vi "Get Position Data.vi"(8 "error in (no error)":errorcluster, 10 "Complete NMEA Sentences":string[](array[string]), 11 "VISA resource name":refnum<visa-resource-name>) -> (0 "error out":errorcluster, 1 "Position Data":T1(array[cluster]), 2 "Complete NMEA Sentences (Copy)":string[](array[string]), 3 "VISA resource name out":refnum<visa-resource-name>)   [LabVIEW 2011, in "u-blox 5 Series.lvlib"]
doc: "Parses out the position data from all of the sentences that Read Raw.vi outputs, and passes through a complete copy of those sentences. Can be used in conjunction with other advanced \"Get\" VIs. See u-blox 5 Series Acquire and Chart GPS Advanced.vi for an example of how to use this VI.\n\nNote that the VISA Resource is not required, since this VI is a helper that does not actually interact with the device. The VISA Resource can be used, however, to clarify programming and maintain uniformity."
uses:
  u-blox 5 Series.lvlib
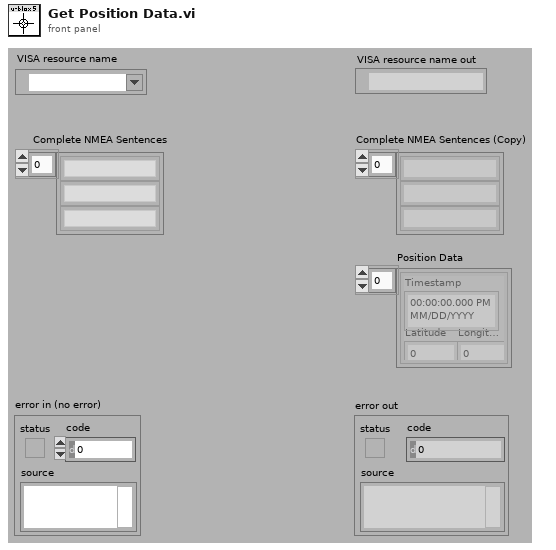
[diagram p1: front panel]
types:
  T1 = cluster{"Timestamp":timestamp, "Latitude":dbl, "Longitude":dbl}[]
  T2 = cluster{"Timestamp":timestamp, "Latitude":dbl, "Longitude":dbl}
  T3 = typedef "u-blox 5 Series.lvlib/GGA Data.ctl" = cluster{"time of fix":cluster{"included?":bool, "time":timestamp}, "latitude":cluster{"included?":bool, "latitude (deg)":dbl}, "longitude":cluster{"included?":bool, "longitude (deg)":dbl}, "fix quality":cluster{"included?":bool, "quality":u16}, "number of satellites in view":cluster{"included?":bool, "number of satellites":i8}, "horizontal dilution of precision":cluster{"included?":bool, "horizontal DOP":dbl}, "altitude above mean sea level":cluster{"included?":bool, "altitude (m)":dbl}, "height of geoid above WGS84":cluster{"included?":bool, "height of geoid (m)":dbl}, "time since last DGPS update":cluster{"included?":bool, "time (s)":dbl}, "DGPS station ID number":cluster{"included?":bool, "station ID number":dbl}}
  T4 = typedef "u-blox 5 Series.lvlib/RMC Data.ctl" = cluster{"time of fix":cluster{"included?":bool, "time":timestamp}, "status":cluster{"included?":bool, "value":u16}, "latitude":cluster{"included?":bool, "latitude (deg)":dbl}, "longitude":cluster{"included?":bool, "longitude (deg)":dbl}, "ground speed":cluster{"included?":bool, "speed (knots)":dbl}, "true track angle":cluster{"included?":bool, "angle (deg)":dbl}, "magnetic variation":cluster{"included?":bool, "variation (deg)":dbl}, "type of fix":cluster{"included?":bool, "mode":u16}}
  T5 = typedef "u-blox 5 Series.lvlib/GLL Data.ctl" = cluster{"latitude":cluster{"included?":bool, "latitude (deg)":dbl}, "longitude":cluster{"included?":bool, "longitude (deg)":dbl}, "time of fix":cluster{"included?":bool, "time":timestamp}, "status":cluster{"included?":bool, "value":u16}, "type of fix":cluster{"included?":bool, "mode":u16}}
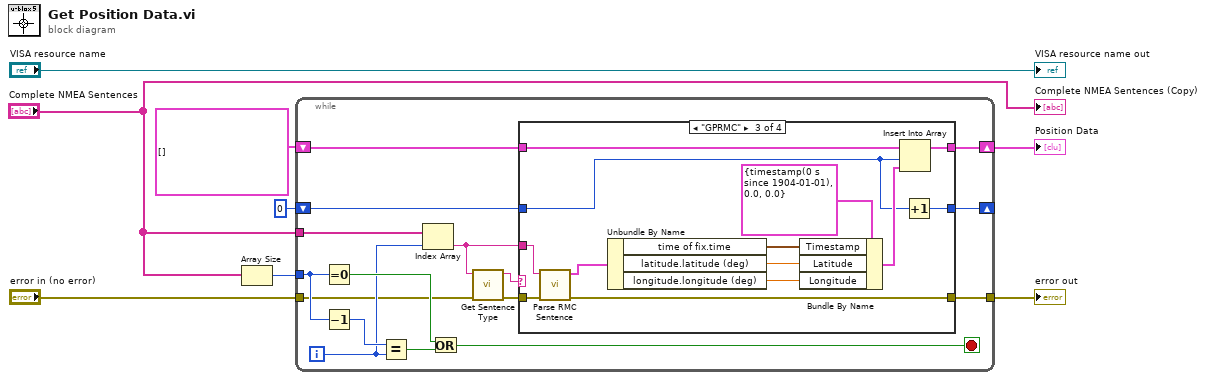
[diagram p0: block diagram]
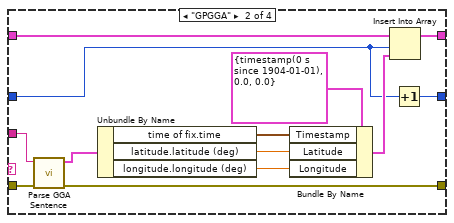
[diagram p3: hidden frame]
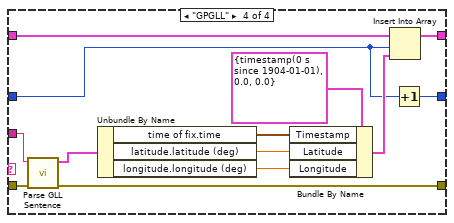
[diagram p4: hidden frame]
diagram:
  n1 = Array Size(array="Complete NMEA Sentences") -> (size(s)=w6:i32)
  n2 = while {
    tunnel: "Complete NMEA Sentences" -> [w24]
    shift-right: [w22] -> w8
    shift-left: T1 [] -> [w21]
    tunnel: w6 -> [w17]
    tunnel: "error in (no error)" -> [w11]
    tunnel: [w23] -> w4
    shift-right: [w19] -> _
    shift-left: 0 -> [w20]
    i -> [w13]
    stop <- w15 stop-if-true
    n3 = Equal To 0?(x=w17) -> (x = 0?=w16:bool)
    n4 = Decrement(x=w17) -> (x-1=w18:i32)
    n5 = Equal?(x=w18, y=w13) -> (x = y?=w14:bool)
    n6 = Index Array(array=w24, index=w13) -> (element=w9:string)
    n7 = Or(x=w16, y=w14) -> (x .or. y?=w15:bool)
    n8 = call "Get Sentence Type.vi"("error in (no error)"=w11, "sentence"=w9) -> ("error out"=w12:errorcluster, "sentence type"=w10:string)  [unwired: 7 in, 1 out]
    n9 = case shown="\"GPRMC\"" w10 {
      tunnel: w9 -> [_ w31 w41 w54]
      tunnel: w12 -> [w27 w29 w43 w56]
      tunnel: [w27 w28 w44 w57] -> w23
      tunnel: [w26 w35 w48 w61] -> w22
      tunnel: w21 -> [w26 w34 w47 w60]
      tunnel: w20 -> [w25 w32 w45 w58]
      tunnel: [w25 w33 w46 w59] -> w19
      frame "", Default {
      }
      frame "GPGGA" {
        n10 = call "Parse GGA Sentence.vi"("error in (no error)"=w29, "GGA sentence"=w31) -> ("error out"=w28:errorcluster, "GGA data"=w30:T3)  [unwired: 8 in]
        n11 = Unbundle By Name(w30) -> ("time of fix.time"=w39:timestamp, "latitude.latitude (deg)"=w38:dbl, "longitude.longitude (deg)"=w37:dbl)
        n12 = Bundle By Name(cluster=T2 {"Timestamp"=timestamp(0 s since 1904-01-01), "Latitude"=0.0, "Longitude"=0.0} ("Cluster"), "Timestamp"=w39, "Latitude"=w38, "Longitude"=w37) -> (w36:T2)
        n13 = Insert Into Array(array=w34, index=w32, new element=w36) -> (w35:T1)
        n14 = Increment(x=w32) -> (x+1=w33:i32)
      }
      frame "GPRMC" {
        n15 = call "Parse RMC Sentence.vi"("error in (no error)"=w43, "RMC sentence"=w41) -> ("error out"=w44:errorcluster, "RMC data"=w42:T4)  [unwired: 8 in]
        n16 = Unbundle By Name(w42) -> ("time of fix.time"=w52:timestamp, "latitude.latitude (deg)"=w51:dbl, "longitude.longitude (deg)"=w50:dbl)
        n17 = Bundle By Name(cluster=T2 {"Timestamp"=timestamp(0 s since 1904-01-01), "Latitude"=0.0, "Longitude"=0.0} ("Cluster"), "Timestamp"=w52, "Latitude"=w51, "Longitude"=w50) -> (w49:T2)
        n18 = Insert Into Array(array=w47, index=w45, new element=w49) -> (w48:T1)
        n19 = Increment(x=w45) -> (x+1=w46:i32)
      }
      frame "GPGLL" {
        n20 = call "Parse GLL Sentence.vi"("error in (no error)"=w56, "GLL sentence"=w54) -> ("error out"=w57:errorcluster, "GLL data"=w55:T5)  [unwired: 8 in]
        n21 = Unbundle By Name(w55) -> ("time of fix.time"=w65:timestamp, "latitude.latitude (deg)"=w64:dbl, "longitude.longitude (deg)"=w63:dbl)
        n22 = Bundle By Name(cluster=T2 {"Timestamp"=timestamp(0 s since 1904-01-01), "Latitude"=0.0, "Longitude"=0.0} ("Cluster"), "Timestamp"=w65, "Latitude"=w64, "Longitude"=w63) -> (w62:T2)
        n23 = Insert Into Array(array=w60, index=w58, new element=w62) -> (w61:T1)
        n24 = Increment(x=w58) -> (x+1=w59:i32)
      }
    }
  }
  "error out" <- w4
  "Position Data" <- w8
  "VISA resource name out" <- "VISA resource name"
  "Complete NMEA Sentences (Copy)" <- "Complete NMEA Sentences"
